vi "Rollers Controller.vi"(8 "error in":errorcluster) -> ()   [LabVIEW 2019]
doc: "This VI executes continuously carrying out the current operation and responding to updates or new operations. It will often contain the timing or control code that is difficult to place directly in TeleOp. This VI generally opens all sensors and motors and isolates the rest of the robot code from knowing how the operations are carried out."
uses:
  <vilib>/Rock Robotics/WPI/Framework/Completion Status.ctl
  Rollers Setpoints.ctl
  Rollers Operations.ctl
  <vilib>/Rock Robotics/WPI/SafetyOutput/WPI_SafetyOutputConfigMenu.ctl
  <vilib>/Rock Robotics/WPI/ThirdParty/REV Robotics/SPARK MAX/Typedef/Spark MAX Control Type.ctl
  <vilib>/addons/control/pid/pid.llb/PID (DBL).vi
  <vilib>/addons/control/pid/NI_PID_pid.lvlib
  <vilib>/Rock Robotics/Network Tables/NT Write Boolean.vi
panel:
  in  "PID gains":T1={"proportional gain (Kc)"=0.1, "integral time (Ti, min)"=0.1, "derivative time (Td, min)"=0.5}
  out "Setpoints":T2(graph)
  in  "Interactive Values":T3
  out "Current\nCmd":string
  in  "Buttons":cluster{"Execute Cmd":bool, "Abort Cmd":bool}
  out "Command Timing":cluster{"Start Time (ms)":u32, "Iterations":i32}
  out "Status":T5
  # "Tip: It may be helpful to observe inputs and sensor values.\nYou may also want to display tuning or debugging controls."
  # "Interactive Command: You may fill in the settings for a command\nand schedule it with the Execute button. You can observe and abort\nany command while fine tuning the code for the controller."
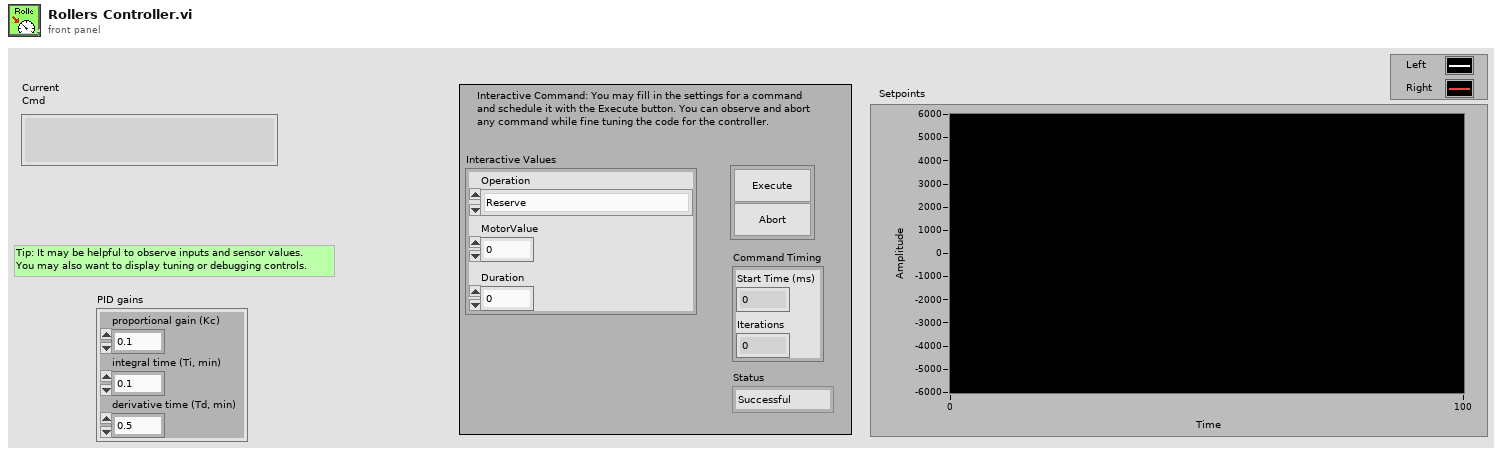
[diagram p1: front panel]
types:
  T1 = cluster{"proportional gain (Kc)":dbl, "integral time (Ti, min)":dbl, "derivative time (Td, min)":dbl}
  T2 = cluster{"Left Setpoint":dbl, "Right Setpoint":dbl}
  T3 = typedef "Rollers Setpoints.ctl" = cluster{"Operation":T4, "MotorValue":dbl, "Duration":dbl}
  T4 = typedef "Rollers Operations.ctl" = enum16{"Reserve", "Read Current", "Immediate", "Roller Duration"}
  T5 = typedef "Completion Status.ctl" = enum16{"Successful", "Aborted", "Incomplete"}
  T6 = typedef "WPI_SafetyOutputConfigMenu.ctl" = enum16{"Enable", "Disable"}
  T7 = typedef "WPI_MotorControlDeviceRef.ctl" = cluster{"DeviceStatus":errorcluster, "Type":T8, "PWM":cluster{"PWM Channel":T9, "DeadBand":T10}, "CAN":cluster{"Device Number":u8, "SetOutput VI Ref":variant, "GetOutput VI Ref":variant, "Enable VI Ref":variant, "Disable VI Ref":variant, "Data":variant}, "Invert":bool, "DIO PWM":cluster{"PWM \"Enable\" Channel":T9, "DIOChannel":T11, "PWM Rate":dbl}}
  T8 = typedef "WPI_MotorControlType.ctl" = enum16{"PWM", "CAN", "DIO PWM"}
  T9 = typedef "FPGA_DIOPWMChannel.ctl" = enum8{"PWM 0", "PWM 1", "PWM 2", "PWM 3", "PWM 4", "PWM 5", "PWM 6", "PWM 7", "PWM 8", "PWM 9", "PWM MXP 0", "PWM MXP 1", "PWM MXP 2", "PWM MXP 3", "PWM MXP 4", "PWM MXP 5", "PWM MXP 6", "PWM MXP 7", "PWM MXP 8", "PWM MXP 9", "Invalid"}
  T10 = typedef "WPI_PWMDeadband.ctl" = cluster{"Name":string, "maxPositivePwm":i32, "minPositivePwm":i32, "centerPwm":i32, "maxNegativePwm":i32, "minNegativePwm":i32, "angularRange":u16}
  T11 = typedef "FPGA_DIOChannel.ctl" = enum8{"DIO 0", "DIO 1", "DIO 2", "DIO 3", "DIO 4", "DIO 5", "DIO 6", "DIO 7", "DIO 8", "DIO 9", "DIO MXP 0", "DIO MXP 1", "DIO MXP 2", "DIO MXP 3", "DIO MXP 4", "DIO MXP 5", "DIO MXP 6", "DIO MXP 7", "DIO MXP 8", "DIO MXP 9", "DIO MXP 10", "DIO MXP 11", "DIO MXP 12", "DIO MXP 13", "DIO MXP 14", "DIO MXP 15", "SPI Port CS1", "SPI Port CS2", "SPI Port CS3", "SPI Port MISO", "SPI Port MOSI", "Invalid"}
  T12 = typedef "Command Status Info.ctl" = cluster{"Name":string, "Status":T5, "notifier out":T13}
  T13 = typedef "Completion Notifier.ctl" = refnum<notifier>
  T14 = cluster{"Current Command":T3, "Command Timing":cluster{"Start Time (ms)":u32, "Iterations":i32}, "Command Arguments":cluster{"Command Info":T12, "Description":string, "Default Command":T3, "queue out":refnum<queue>, "Subsystem Name":string}}
  T15 = typedef "Spark MAX Control Type.ctl" = enum16{"Percent VBus", "Voltage", "Velocity", "Position", "Smart Motion", "Current", "Smart Velocity"}
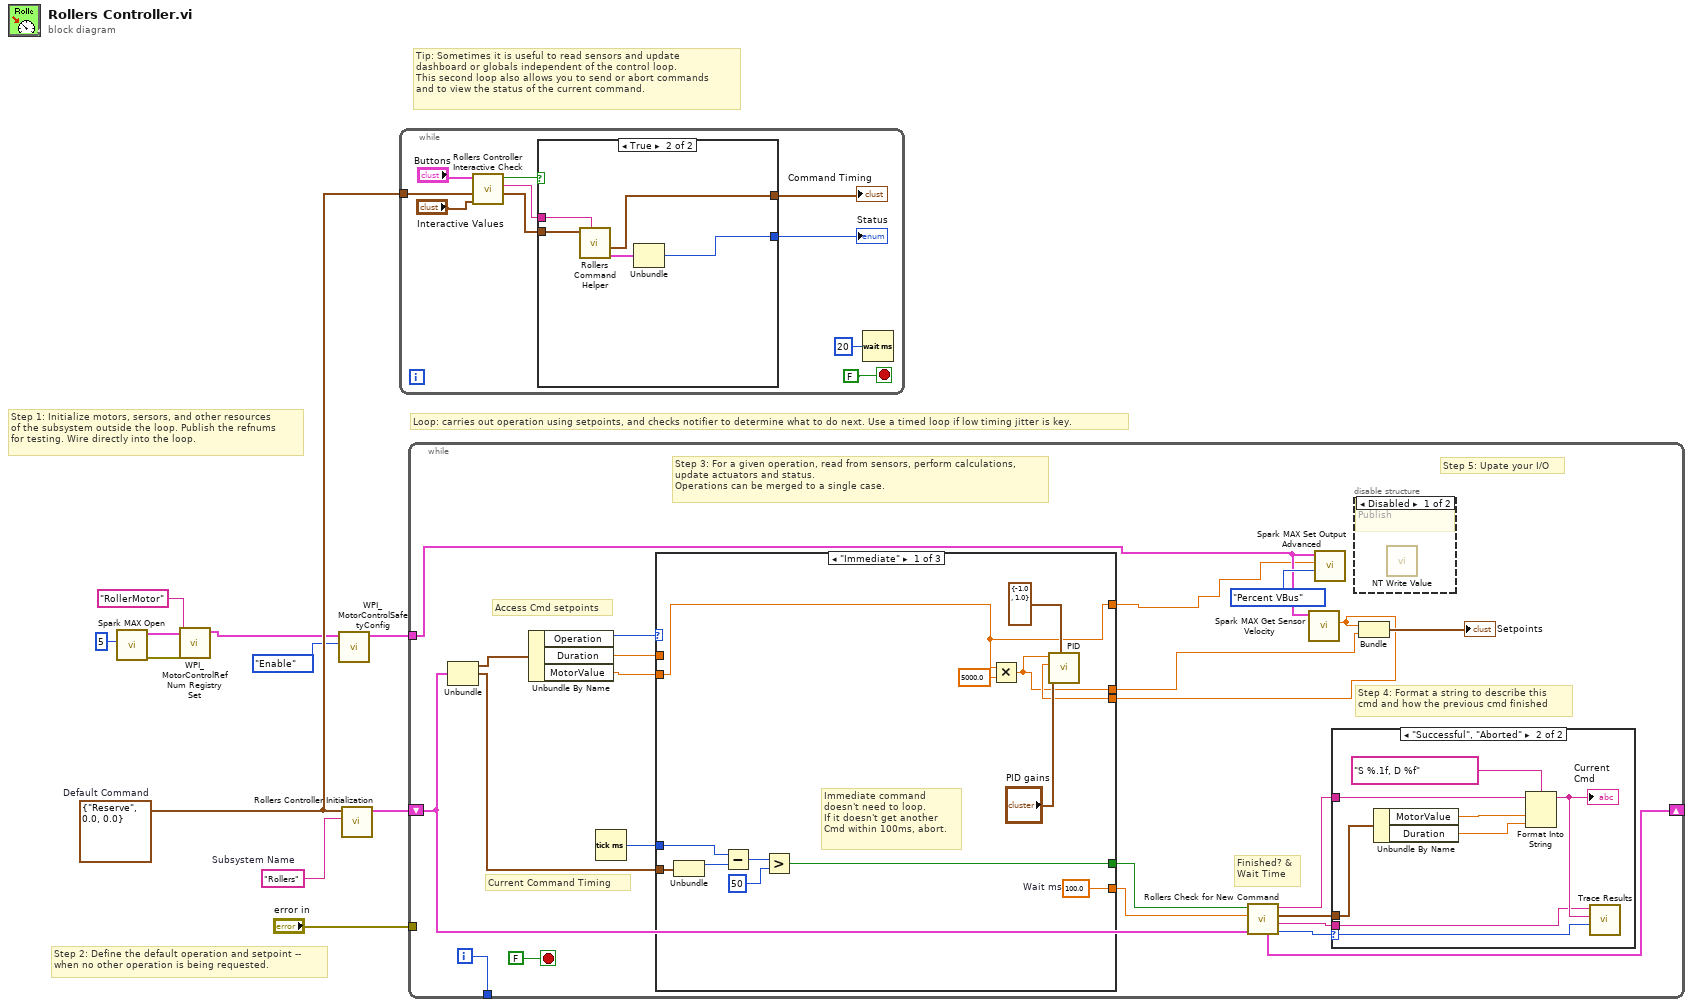
[diagram p0: block diagram]
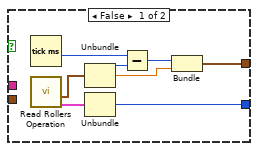
[diagram p2: hidden frame]
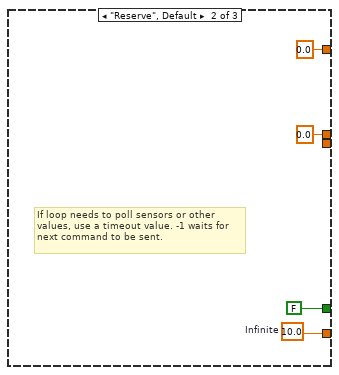
[diagram p5: hidden frame]
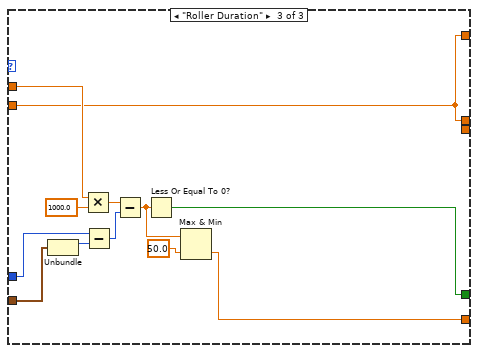
[diagram p6: hidden frame]
diagram:
  w8 = T3 {"Operation"=enum."Reserve", "MotorValue"=0.0, "Duration"=0.0}  # Default Command
  w9 = "Rollers"  # Subsystem Name
  # "Tip: Sometimes it is useful to read sensors and update\ndashboard or globals independent of the control loop.\nThis second loop also allows you to send or abort commands\nand to view the status of the current command."
  # "Step 2: Define the default operation and setpoint --\nwhen no other operation is being requested."
  # "Step 1: Initialize motors, sersors, and other resources\nof the subsystem outside the loop. Publish the refnums\nfor testing. Wire directly into the loop."
  # "Loop: carries out operation using setpoints, and checks notifier to determine what to do next. Use a timed loop if low timing jitter is key."
  n1 = call <vilib>:"Spark MAX Open.vi"("Device Number"=u8 5) -> ("error out"=w1:errorcluster, "MotorControlDeviceRef"=w7:T7)  [unwired: 9 in]
  n2 = call <vilib>:"WPI_MotorControlRefNum Registry Set.vi"("error in (no error)"=w1, "refnum name"="RollerMotor", "MotorControlDevRef"=w7) -> ("MotorControlDevRef"=w5:T7)  [unwired: 7 in, 1 out]
  n3 = call <vilib>:"WPI_MotorControlSafetyConfig.vi"("mode"=WPI_SafetyOutputConfigMenu."Enable", "MotorControlDevRef"=w5) -> ("MotorControlDevRef"=w3:T7)  [unwired: 8 in, 1 out]
  n4 = call "Rollers Controller Initialization.vi"("Subsystem Name"=w9, "Default Command"=w8) -> ("Current Command"=w10:T14)  [unwired: 9 in]
  n5 = while {
    tunnel: w8 -> [w18]
    stop <- FALSE stop-if-true
    n6 = call "Rollers Controller Interactive Check.vi"("Interactive Command in"="Interactive Values", "Default Command"=w18, "Buttons"="Buttons") -> ("Interactive Command out"=w15:T3, "Trace String"=w16:string, "Schedule"=w17:bool)  [unwired: 6 in]
    n7 = case shown="True" w17 {
      tunnel: [w29 w34] -> w14
      tunnel: w15 -> [_ w32]
      tunnel: [w25 w30] -> w13
      tunnel: w16 -> [_ w33]
      frame False {
        n8 = Tick Count (ms)() -> (millisecond timer value=w24:u32)
        n9 = call "Read Rollers Operation.vi"() -> ("Command Info"=w22:T12, "SubSystem Data"=w23:T3)  [unwired: 9 in, 1 out]
        n10 = Unbundle(w23) -> ("Operation"=w28:T4, "MotorValue"=w26:dbl)  [unwired: 1 out]
        n11 = Unbundle(w22) -> ("Status"=w29:T5)  [unwired: 2 out]
        n12 = Subtract(x=w24, y=w28) -> (x-y=w27:u32)
        n13 = Bundle(w27, "MotorValue"=w26) -> (w25:cluster{u32, "MotorValue":dbl})  [unwired: 1 in]
      }
      frame True {
        n14 = call "Rollers Command Helper.vi"("Description"=w33, "SubSystem Data"=w32) -> ("Command Info Out"=w31:T12, "Command Timing"=w30:cluster{"Start Time (ms)":u32, "Iterations":i32})  [unwired: 7 in, 1 out]
        n15 = Unbundle(w31) -> ("Status"=w34:T5)  [unwired: 2 out]
      }
    }
    "Status" <- w14
    "Command Timing" <- w13
    n16 = Wait (ms)(milliseconds to wait=u32 20) -> ()  [unwired: 1 out]
  }
  n17 = while {
    shift-right: [w48] -> _
    shift-left: w10 -> [w41]
    tunnel: [w55] -> _
    tunnel: "error in" -> [_]
    tunnel: w3 -> [w38]
    i -> [w55]
    stop <- FALSE stop-if-true
    # "Step 5: Upate your I/O"
    # "Step 4: Format a string to describe this\ncmd and how the previous cmd finished"
    # "Current Command Timing"
    # "Access Cmd setpoints"
    # "Finished? &\nWait Time"
    # "Step 3: For a given operation, read from sensors, perform calculations,\nupdate actuators and status.\nOperations can be merged to a single case."
    n18 = Unbundle(w41) -> ("Current Command"=w54:T3, "Command Timing"=w50:cluster{"Start Time (ms)":u32, "Iterations":i32})  [unwired: 1 out]
    n19 = Unbundle By Name(w54) -> ("Operation"=w53:T4, "Duration"=w52:dbl, "MotorValue"=w49:dbl)
    n20 = Tick Count (ms)() -> (millisecond timer value=w51:u32)
    n21 = call <vilib>:"Spark MAX Get Sensor Velocity.vi"("MotorControlDevRef in"=w38) -> ("Sensor Velocity"=w35:dbl)  [unwired: 7 in, 3 out]
    n22 = case shown="\"Immediate\"" w53 {
      tunnel: [w77 w81 w83] -> w46
      tunnel: [w71 FALSE ("ignore previous (F)") w84] -> w47
      tunnel: w50 -> [w73 _ w87]
      tunnel: w52 -> [_ _ w85]
      tunnel: w51 -> [w72 _ w86]
      tunnel: w49 -> [w65 _ w82]
      tunnel: [w65 0.0 ("MotorValue") w82] -> w37
      tunnel: w35 -> [w68 _ _]
      tunnel: [w66 0.0 w82] -> w36
      frame "Immediate" {
        w77 = 100.0  # Wait ms
        # "Immediate command\ndoesn't need to loop.\nIf it doesn't get another\nCmd within 100ms, abort."
        n23 = Unbundle(w73) -> ("Start Time (ms)"=w76:u32)  [unwired: 1 out]
        n24 = Subtract(x=w72, y=w76) -> (x-y=w75:u32)
        n25 = Greater?(x=w75, y=u8 50 ("Left Motor")) -> (0:w71:bool)
        n26 = Multiply(x=w65, y=5000.0) -> (x*y=w66:dbl)
        n27 = call-poly <vilib>:"PID.vi"("output range"=cluster{"output low":dbl, "output high":dbl} {"output low"=-1.0, "output high"=1.0}, "PID gains"="PID gains", "process variable"=w68, "setpoint"=w66) -> ()  [unwired: 6 in, 2 out]
      }
      frame "Reserve", Default {
        w81 = 10.0  # Infinite
        # "If loop needs to poll sensors or other\nvalues, use a timeout value. -1 waits for\nnext command to be sent."
      }
      frame "Roller Duration" {
        n28 = Unbundle(w87) -> ("Start Time (ms)"=w90:u32)  [unwired: 1 out]
        n29 = Multiply(x=w85, y=1000.0) -> (x*y=w92:dbl)
        n30 = Subtract(x=w86, y=w90) -> (x-y=w93:u32)
        n31 = Subtract(x=w92, y=w93) -> (x-y=w89:dbl)
        n32 = Less Or Equal To 0?(x=w89) -> (x <= 0?=w84:bool)
        n33 = Max & Min(x=w89, y=50.0) -> (min(x,y)=w83:dbl)  [unwired: 1 out]
      }
    }
    n34 = call "Rollers Check for New Command.vi"("Current Command"=w41, "Wait time (ms)"=w46, "Finished?"=w47) -> ("Completion"=w42:T5, "Subsystem Name"=w43:string, "Current Command"=w44:T3, "Initial Trace String"=w45:string, "NextCommand"=w48:T14)  [unwired: 4 in]
    n35 = call <vilib>:"Spark MAX Set Output Advanced.vi"("Control Mode"=Spark_MAX_Control_Type."Percent VBus", "Setpoint"=w37, "MotorControlDevRef"=w38) -> ()  [unwired: 7 in, 2 out]
    n36 = case shown="\"Successful\", \"Aborted\"" w42 {
      selector: w42 -> [_ w64]
      tunnel: w45 -> [_ w60]
      tunnel: w44 -> [_ w61]
      tunnel: w43 -> [_ w57]
      frame "Incomplete", Default {
        # "Continuing current command"
      }
      frame "Successful", "Aborted" {
        # "Report and setup for next command"
        n37 = Unbundle By Name(w61) -> ("MotorValue"=w63:dbl, "Duration"=w58:dbl)
        n38 = Format Into String(format string="S %.1f, D %f", initial string=w60, w63, w58) -> (resulting string=w59:string)  [unwired: 1 in, 1 out]
        "Current\nCmd" <- w59
        n39 = call <vilib>:"Trace Results.vi"("Status of previous command"=w64, "Description"=w59, "Subsystem"=w57) -> ()  [unwired: 9 in]
      }
    }
    n40 = disable-structure shown="Disabled" {
      frame Disabled {
        # "Publish"
        n41 = call-poly <vilib>:"NT Write Value.vi"() -> ()  [unwired: 11 in, 1 out]
      }
      frame Enabled {
      }
    }
    n42 = Bundle("Sensor Velocity"=w35, "MotorValue"=w36) -> (→"Setpoints":cluster{"Sensor Velocity":dbl, "MotorValue":dbl})  [unwired: 1 in]
  }
